vi "VFH Visualization.vi"() -> (0 "Heading History":dbl(graph), 1 "VY History":dbl(graph), 3 "LIDAR data":cluster{dbl[], dbl[]}[](graph))   [LabVIEW 2018]
uses:
  <vilib>/Analysis/coordinate.llb/Wrap Angle (scalar).vi
  <vilib>/Analysis/coordinate.llb/2D Cartesian Coordinate Rotation (Array).vi
  <vilib>/Analysis/NI_AALPro.lvlib
  <vilib>/Analysis/NI_AAL_Angle.lvlib
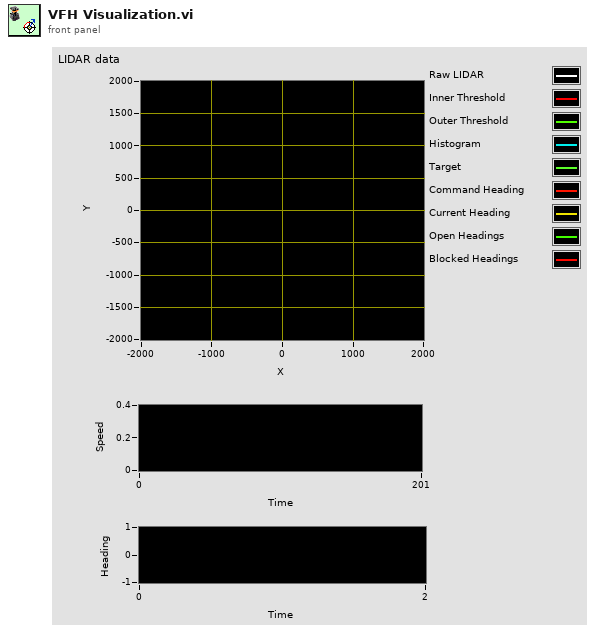
[diagram p1: front panel]
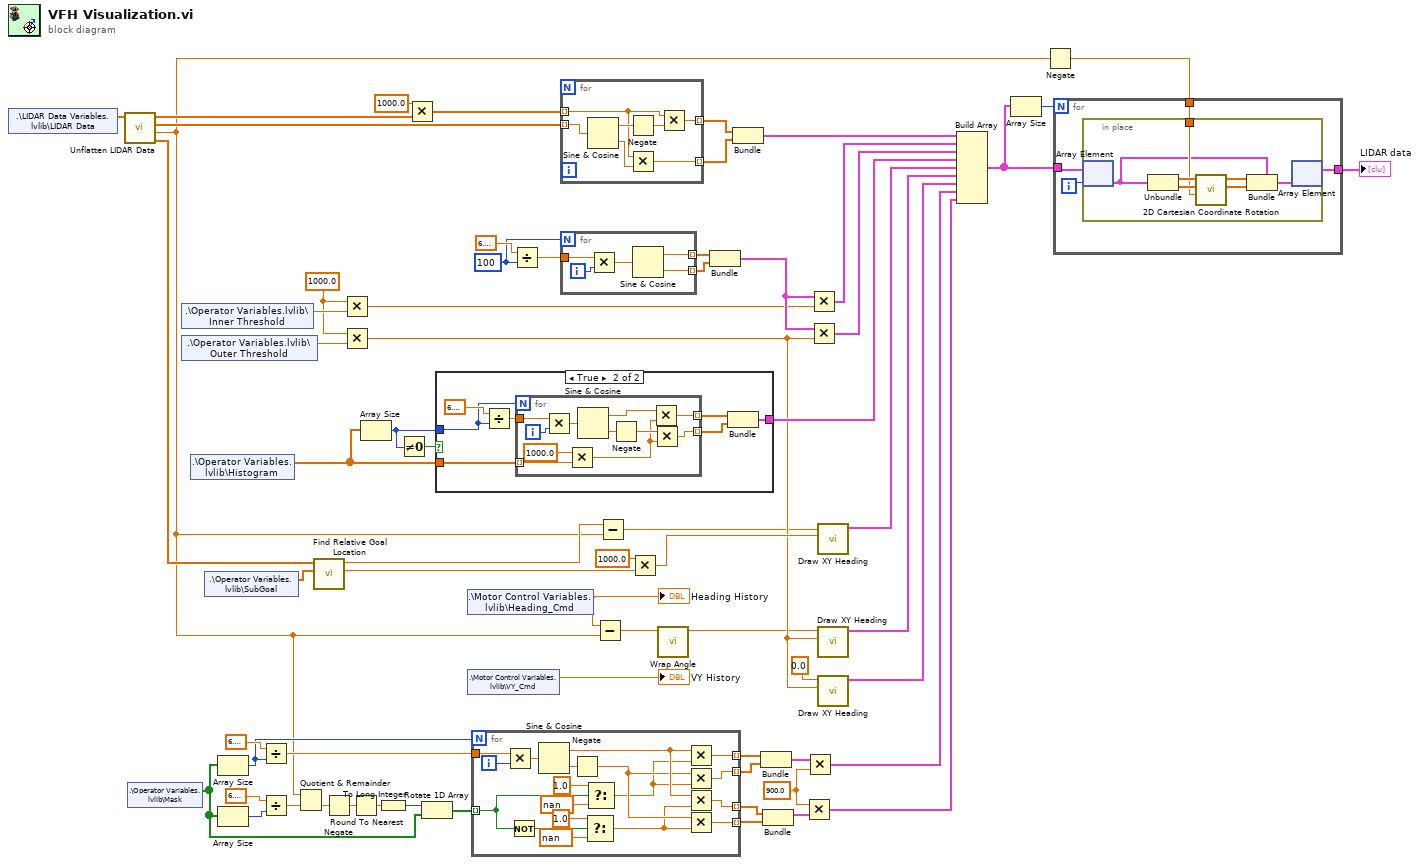
[diagram p0: block diagram]
diagram:
  w17 = 1000.0 ("x")
  w3 = 900.0 ("y")
  w64 = 100 ("y")
  n1 = shared-variable ".\\LIDAR Data Variables.lvlib\\LIDAR Data"() -> (w15:dbl[])  [unwired: 1 in, 1 out]
  n2 = call "Unflatten LIDAR Data.vi"("Flat LIDAR Data"=w15) -> ("Robot Pose x,y (m)"=w12:dbl[], "Robot Pose Theta (rad)"=w8:dbl, "Bearing (rad)"=w13:dbl[], "Range (m)"=w14:dbl[])  [unwired: 7 in]
  n3 = shared-variable ".\\Operator Variables.lvlib\\Mask"() -> (w33:bool[])  [unwired: 1 in, 1 out]
  n4 = shared-variable ".\\Operator Variables.lvlib\\Inner Threshold"() -> (w22:dbl)  [unwired: 1 in, 1 out]
  n5 = shared-variable ".\\Operator Variables.lvlib\\Outer Threshold"() -> (w21:dbl)  [unwired: 1 in, 1 out]
  n6 = shared-variable ".\\Operator Variables.lvlib\\Histogram"() -> (w38:dbl[])  [unwired: 1 in, 1 out]
  n7 = shared-variable ".\\Operator Variables.lvlib\\SubGoal"() -> (w37:dbl[])  [unwired: 1 in, 1 out]
  n8 = Array Size(array=w33) -> (size(s)=w56:i32)
  n9 = Array Size(array=w33) -> (size(s)=w48:i32)
  n10 = Divide(x=6.283185307179586, y=w56) -> (x/y=w57:dbl)
  n11 = Divide(x=6.283185307179586, y=w48) -> (x/y=w47:dbl)
  n12 = Quotient & Remainder(x=w8, y=w47) -> (floor(x/y)=w46:dbl)  [unwired: 1 out]
  n13 = call "Find Relative Goal Location.vi"("Goal Position"=w37, "Current Position"=w12) -> ("Target Distance"=w34:dbl, "Target Heading"=w9:dbl)  [unwired: 8 in]
  n14 = Negate(x=w46) -> (-x=w45:dbl)
  n15 = Multiply(x=w17, y=w22) -> (x*y=w19:dbl)
  n16 = Multiply(x=w17, y=w21) -> (x*y=w18:dbl)
  n17 = Round To Nearest(number=w45) -> (nearest integer value=w44:dbl)
  n18 = Array Size(array=w38) -> (size(s)=w32:i32)
  n19 = To Long Integer(number=w44) -> (32bit integer=w43:i32)
  n20 = Not Equal To 0?(x=w32) -> (x != 0?=w31:bool)
  n21 = Multiply(x=1000.0, y=w14) -> (x*y=w11:dbl[])
  n22 = Rotate 1D Array(1:w33, 2:w43) -> (0:w42:bool[])
  n23 = case shown="True" w31 {
    tunnel: [_ w73] -> w30
    tunnel: w38 -> [_ w68]
    tunnel: w32 -> [_ w67]
    frame False {
    }
    frame True {
      n24 = Divide(x=6.283185307179586, y=w67) -> (x/y=w70:dbl)
      n25 = for {
        N: w67 -> [_]
        tunnel: w70 -> [w83]
        tunnel: [w78] -> w71 mode=indexing
        tunnel: [w77] -> w72 mode=indexing
        tunnel: w68 -> [w76] mode=indexing
        i -> [w84]
        n26 = Multiply(x=w83, y=w84) -> (x*y=w82:dbl)
        n27 = Multiply(x=1000.0, y=w76) -> (x*y=w75:dbl)
        n28 = Sine & Cosine(0:w82) -> (1:w81:dbl, 2:w80:dbl)
        n29 = Negate(x=w80) -> (-x=w79:dbl)
        n30 = Multiply(x=w81, y=w75) -> (x*y=w78:dbl)
        n31 = Multiply(x=w79, y=w75) -> (x*y=w77:dbl)
      }
      n32 = Bundle(w71, w72) -> (w73:cluster{dbl[], dbl[]})  [unwired: 1 out]
    }
  }
  n33 = shared-variable ".\\Motor Control Variables.lvlib\\Heading_Cmd"() -> (w24:dbl)  [unwired: 1 in, 1 out]
  "Heading History" <- w24
  n34 = shared-variable ".\\Motor Control Variables.lvlib\\VY_Cmd"() -> (→"VY History":dbl)  [unwired: 1 in, 1 out]
  n35 = for {
    N: w56 -> [_]
    tunnel: w57 -> [w101]
    tunnel: [w92] -> w54 mode=indexing
    tunnel: [w91] -> w53 mode=indexing
    tunnel: w42 -> [w94] mode=indexing
    tunnel: [w89] -> w52 mode=indexing
    tunnel: [w90] -> w51 mode=indexing
    i -> [w102]
    n36 = Multiply(x=w101, y=w102) -> (x*y=w100:dbl)
    n37 = Not(x=w94) -> (.not. x?=w93:bool)
    n38 = Sine & Cosine(0:w100) -> (1:w88:dbl, 2:w99:dbl)
    n39 = Negate(x=w99) -> (-x=w87:dbl)
    n40 = Select(t=1.0, s=w93, f=nan) -> (s? t:f=w85:dbl)
    n41 = Select(t=1.0, s=w94, f=nan) -> (s? t:f=w86:dbl)
    n42 = Multiply(x=w88, y=w86) -> (x*y=w92:dbl)
    n43 = Multiply(x=w87, y=w86) -> (x*y=w91:dbl)
    n44 = Multiply(x=w88, y=w85) -> (x*y=w89:dbl)
    n45 = Multiply(x=w87, y=w85) -> (x*y=w90:dbl)
  }
  n46 = Divide(x=6.283185307179586, y=w64) -> (x/y=w63:dbl)
  n47 = for {
    tunnel: w11 -> [w103] mode=indexing
    tunnel: w13 -> [w104] mode=indexing
    tunnel: [w107] -> w39 mode=indexing
    tunnel: [w106] -> w40 mode=indexing
    n48 = Sine & Cosine(0:w104) -> (1:w109:dbl, 2:w108:dbl)
    n49 = Negate(x=w109) -> (-x=w105:dbl)
    n50 = Multiply(x=w103, y=w108) -> (x*y=w106:dbl)
    n51 = Multiply(x=w103, y=w105) -> (x*y=w107:dbl)
  }
  n52 = for {
    N: w64 -> [_]
    tunnel: w63 -> [w113]
    tunnel: [w111] -> w62 mode=indexing
    tunnel: [w110] -> w61 mode=indexing
    i -> [w114]
    n53 = Multiply(x=w113, y=w114) -> (x*y=w112:dbl)
    n54 = Sine & Cosine(0:w112) -> (1:w111:dbl, 2:w110:dbl)
  }
  n55 = Subtract(x=w24, y=w8) -> (x-y=w2:dbl)
  n56 = Subtract(x=w9, y=w8) -> (x-y=w7:dbl)
  n57 = Multiply(x=1000.0 ("y"), y=w34) -> (x*y=w35:dbl)
  n58 = call-poly <vilib>:"Wrap Angle.vi"("angle in"=w2) -> ("angle out"=w1:dbl)  [unwired: 9 in, 1 out]
  n59 = Bundle(w62, w61) -> (w20:cluster{dbl[], dbl[]})  [unwired: 1 out]
  n60 = Bundle(w39, w40) -> (w66:cluster{dbl[], dbl[]})  [unwired: 1 out]
  n61 = Bundle(w54, w53) -> (w55:cluster{dbl[], dbl[]})  [unwired: 1 out]
  n62 = Bundle(w52, w51) -> (w50:cluster{dbl[], dbl[]})  [unwired: 1 out]
  n63 = Multiply(x=w3, y=w50) -> (x*y=w25:cluster{dbl[], dbl[]})
  n64 = Multiply(x=w55, y=w3) -> (x*y=w26:cluster{dbl[], dbl[]})
  n65 = Multiply(x=w20, y=w19) -> (x*y=w23:cluster{dbl[], dbl[]})
  n66 = Multiply(x=w20, y=w18) -> (x*y=w60:cluster{dbl[], dbl[]})
  n67 = call "Draw XY Heading.vi"("Length"=w35, "Direction"=w7) -> ("Heading Graph"=w29:cluster{dbl[], dbl[]})  [unwired: 9 in]
  n68 = call "Draw XY Heading.vi"("Length"=w18, "Direction"=w1) -> ("Heading Graph"=w28:cluster{dbl[], dbl[]})  [unwired: 9 in]
  n69 = call "Draw XY Heading.vi"("Length"=w18, "Direction"=0.0) -> ("Heading Graph"=w27:cluster{dbl[], dbl[]})  [unwired: 9 in]
  n70 = Build Array(w66, w23, w60, w30, w29, w28, w27, w26, w25) -> (w5:cluster{dbl[], dbl[]}[])
  n71 = Array Size(array=w5) -> (size(s)=w4:i32)
  n72 = Negate(x=w8) -> (-x=w59:dbl)
  n73 = for {
    N: w4 -> [_]
    tunnel: w5 -> [w117]
    tunnel: w59 -> [w118]
    tunnel: [w116] -> w6
    i -> [w115]
    n74 = in-place {
      in-place-border: w118 -> [w121]
      n75 = in-place-array #1(w117, w115) -> (w120:cluster{dbl[], dbl[]})
      n76 = Unbundle(w120) -> (w125:dbl[], w124:dbl[])
      n77 = call-poly <vilib>:"2D Cartesian Coordinate Rotation.vi"("theta"=w121, "Y"=w124, "X"=w125) -> ("Y Out"=w122:dbl[], "X Out"=w123:dbl[])  [unwired: 6 in, 1 out]
      n78 = Bundle(cluster=w120, w123, w122) -> (w119:cluster{dbl[], dbl[]})
      n79 = in-place-array #1(w119) -> (w116:cluster{dbl[], dbl[]}[])  [unwired: 1 out]
    }
  }
  "LIDAR data" <- w6
